vi "Add_Vectors_R_Theta.vi"(8 "theta2(rad)":dbl, 9 "r2":dbl, 10 "theta1(rad)":dbl, 11 "r1":dbl) -> (1 "theta3(rad)":dbl, 2 "r3":dbl)   [LabVIEW 2019]
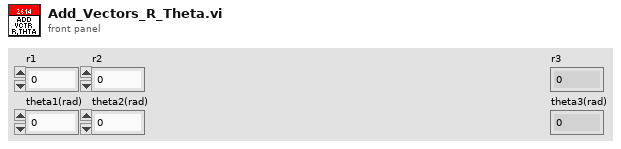
[diagram p1: front panel]
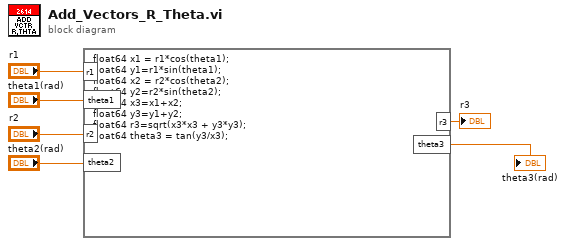
[diagram p0: block diagram]
diagram:
  n1 = formula code="float64 x1 = r1*cos(theta1);\nfloat64 y1=r1*sin(theta1);\nfloat64 x2 = r2*cos(theta2);\nfloat64 y2=r2*sin(theta2);\nfloat64 x3=x1+x2;\nfloat64 y3=y1+y2;\nfloat64 r3=sqrt(x3*x3 + y3*y3);\nfloat64 theta3 = tan(y3/x3);"("r1"="r1", "theta1"="theta1(rad)", "r2"="r2", "theta2"="theta2(rad)") -> ("theta3"=→"theta3(rad)":dbl, "r3"=→"r3":dbl)
